vi "Renumber.vi"(8 "Error In":errorcluster, 10 "Value":dbl, 11 "Thorlabs in":refnum<class "Thorlabs.lvclass">) -> (0 "Error Out":errorcluster, 3 "Thorlabs out":refnum<class "Thorlabs.lvclass">)   [LabVIEW 2018, in "Thorlabs.lvlib" / "Thorlabs.lvclass"]
uses:
  Thorlabs.lvclass
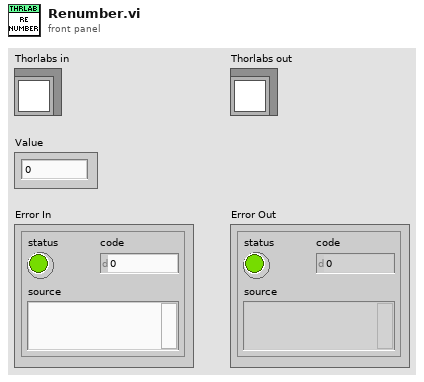
[diagram p1: front panel]
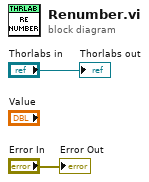
[diagram p0: block diagram]
diagram:
  "Thorlabs out" <- "Thorlabs in"
  "Error Out" <- "Error In"
